vi "Shoot Low Goal State Machine.vi"   [LabVIEW 2013]
uses:
  typedefs/singleUseSubstate.ctl
  typedefs/subStates.ctl
panel:
  # "A State Machine to Handle a Low Goal Shot"
types:
  T1 = typedef "singleUseSubstate.ctl" = enum16{"null", "wait", "shift high", "shift low", "cock shooter", "retract shooter", "latch", "unlatch"}
  T2 = typedef "subStates.ctl" = enum16{"null", "wait", "driver control", "auto", "manual override", "hold position", "rotate", "pickup", "pass", "load", "goto shoot", "shoot high goal", "shoot low goal", "cancel arm", "cancel shooter", "end"}
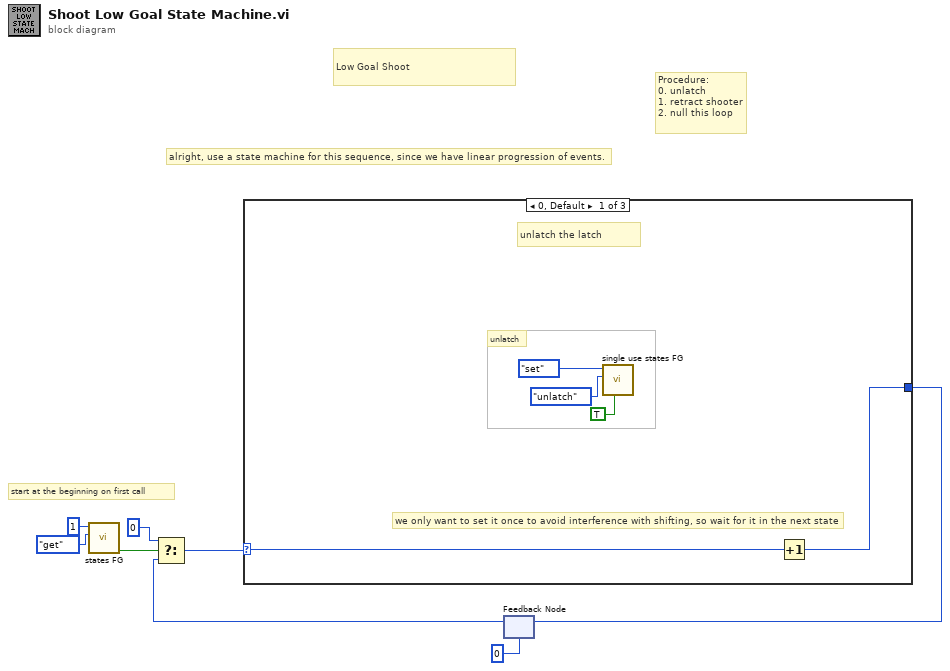
[diagram p0: block diagram]
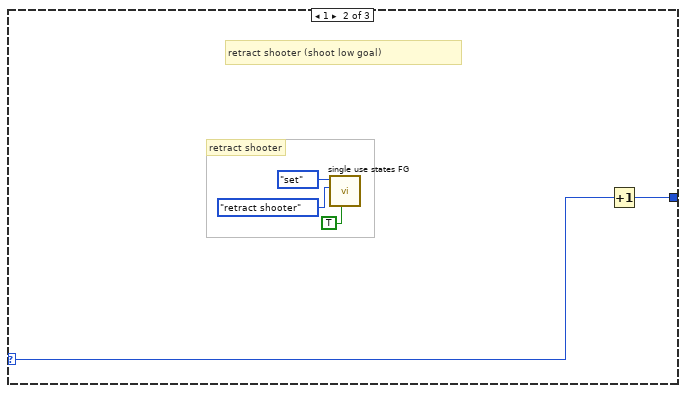
[diagram p2: hidden frame]
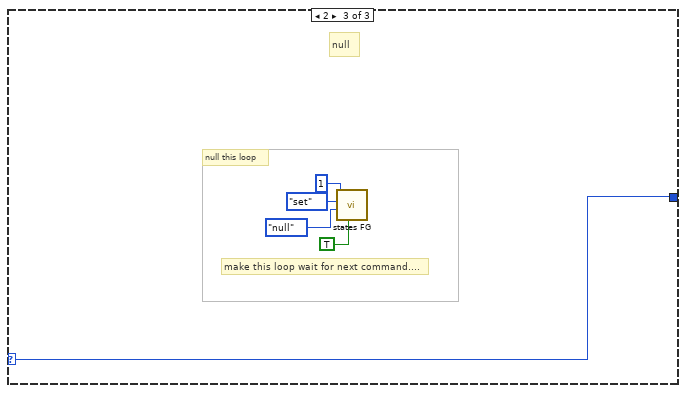
[diagram p3: hidden frame]
diagram:
  # "start at the beginning on first call"
  # "Low Goal Shoot"
  # "Procedure: \n0. unlatch\n1. retract shooter\n2. null this loop"
  # "alright, use a state machine for this sequence, since we have linear progression of events."
  n1 = call "states FG.vi"("menu (get)"=enum16{"set", "get"}."get", "Loop ID"=1) -> ("first call?"=w1:bool)  [unwired: 6 in, 3 out]
  n2 = feedback #1(u8 0) -> (w4:u8)
  n3 = Select(t=u8 0, s=w1, f=w4) -> (s? t:f=w3:u8)
  n4 = case shown="0, Default" w3 {
    selector: w3 -> [w13 w18 w23]
    tunnel: [w12 w17 w23] -> w7
    frame 0, Default {
      # "we only want to set it once to avoid interference with shifting, so wait for it in the next state"
      # "unlatch the latch"
      # "unlatch"
      n5 = call "single use states FG.vi"("exit in"=TRUE, "substate"=singleUseSubstate."unlatch", "menu (get)"=enum16{"set", "get"}."set") -> ()  [unwired: 5 in, 4 out]
      n6 = Increment(x=w13) -> (x+1=w12:u8)
    }
    frame 1 {
      # "retract shooter"
      # "retract shooter (shoot low goal)"
      n7 = call "single use states FG.vi"("exit in"=TRUE, "substate"=singleUseSubstate."retract shooter", "menu (get)"=enum16{"set", "get"}."set") -> ()  [unwired: 5 in, 4 out]
      n8 = Increment(x=w18) -> (x+1=w17:u8)
    }
    frame 2 {
      # "null this loop"
      # "make this loop wait for next command...."
      # "null"
      n9 = call "states FG.vi"("exit in"=TRUE, "subState in"=subStates."null", "menu (get)"=enum16{"set", "get"}."set", "Loop ID"=1) -> ()  [unwired: 4 in, 4 out]
    }
  }
  n10 = feedback-in #1(w7) -> ()
